vi "get pn type.vi"(11 "字符串":string) -> (1 "type adder":string, 3 "type":i32)   [LabVIEW 2011]
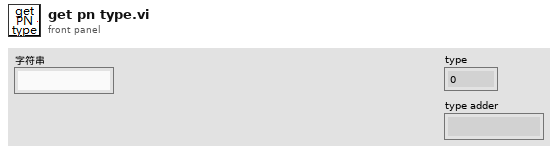
[diagram p1: front panel]
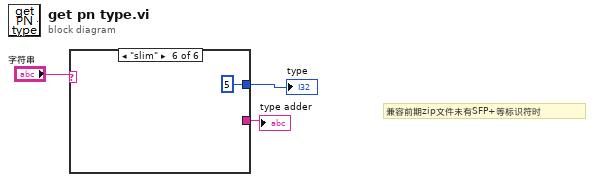
[diagram p0: block diagram]
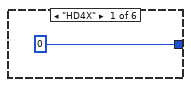
[diagram p2: hidden frame]
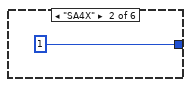
[diagram p3: hidden frame]
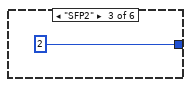
[diagram p4: hidden frame]
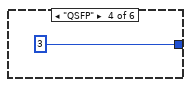
[diagram p5: hidden frame]
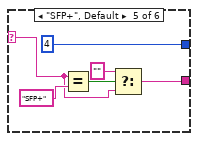
[diagram p6: hidden frame]
diagram:
  # "兼容前期zip文件未有SFP+等标识符时"
  n1 = case shown="\"slim\"" "字符串" {
    selector: "字符串" -> [_ _ _ _ w10 _]
    tunnel: [0 1 2 3 4 5] -> w2
    tunnel: [_ _ _ _ w8 _] -> w1
    frame "HD4X" {
    }
    frame "SA4X" {
    }
    frame "SFP2" {
    }
    frame "QSFP" {
    }
    frame "SFP+", Default {
      n2 = Equal?(x=w10, y="SFP+") -> (x = y?=w11:bool)
      n3 = Select(t="", s=w11, f=w10) -> (s? t:f=w8:string)
    }
    frame "slim" {
    }
  }
  "type" <- w2
  "type adder" <- w1
